vi "BypassControl.vi"(6 "Cutoff":dbl=0.15 format="%#_13g", 8 "MaxMotorChangeForward":dbl, 9 "MaxMotorChangeBackward":dbl, 10 "DesiredInput":dbl, 11 "CurrentInput":dbl) -> (2 "In range?":bool, 3 "SetMotor":dbl)   [LabVIEW 2015]
doc: "Skips motor values that are, for all intents and purposes, 0. This VI includes trapezoidal acceleration."
panel:
  in  "LoopTime":dbl
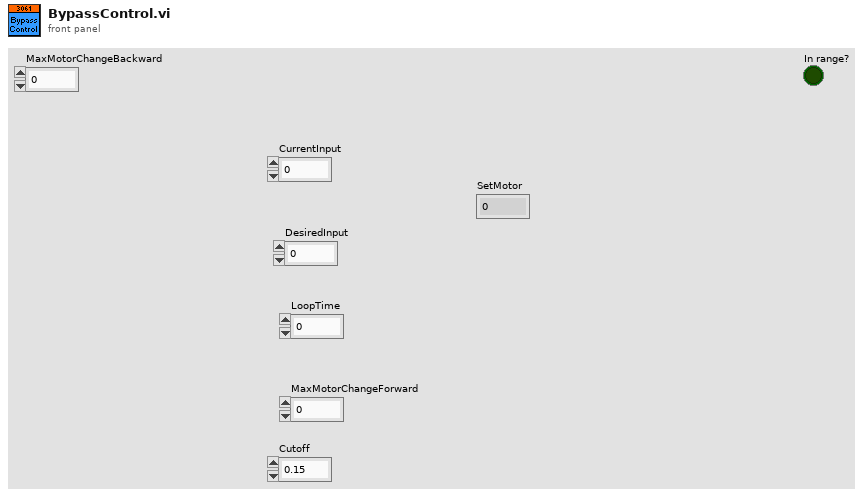
[diagram p1: front panel]
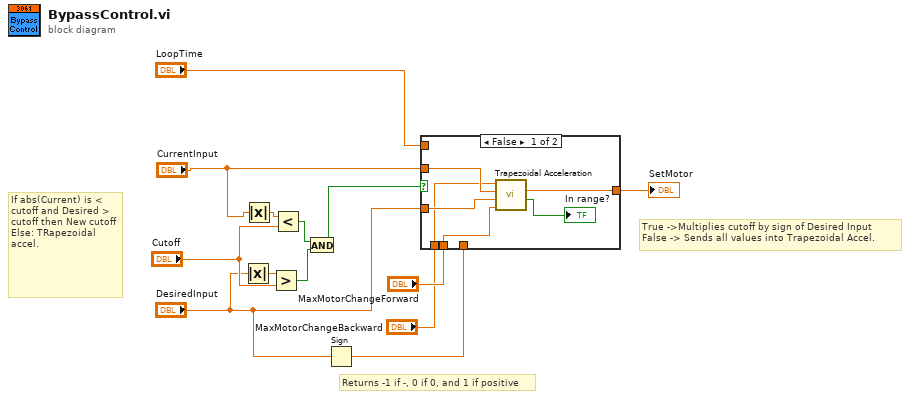
[diagram p0: block diagram]
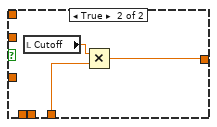
[diagram p2: hidden frame]
diagram:
  # "If abs(Current) is < cutoff and Desired > cutoff then New cutoff\nElse: TRapezoidal accel."
  # "True ->Multiplies cutoff by sign of Desired Input \nFalse -> Sends all values into Trapezoidal Accel."
  # "Returns -1 if -, 0 if 0, and 1 if positive"
  n1 = Absolute Value(x="DesiredInput") -> (abs(x)=w11:dbl)
  n2 = Absolute Value(x="CurrentInput") -> (abs(x)=w12:dbl)
  n3 = Greater?(x=w11, y="Cutoff") -> (0:w9:bool)
  n4 = Less?(x=w12, y="Cutoff") -> (x < y?=w10:bool)
  n5 = And(x=w10, y=w9) -> (x .and. y?=w8:bool)
  n6 = Sign(1:"DesiredInput") -> (0:w6:dbl)
  n7 = case shown="False" w8 {
    tunnel: "DesiredInput" -> [w18 _]
    tunnel: "CurrentInput" -> [w19 _]
    tunnel: [w17 w22] -> w5
    tunnel: w6 -> [_ w21]
    tunnel: "LoopTime" -> [_ _]
    tunnel: "MaxMotorChangeForward" -> [w16 _]
    tunnel: "MaxMotorChangeBackward" -> [w14 _]
    frame False {
      n8 = call "Trapezoidal Acceleration.vi"("MaxMotorChangeForward"=w16, "Desired"=w18, "Actual"=w19, "MaxMotorChangeBackward"=w14) -> ("In range?"=→"In range?":bool, "New Actual"=w17:dbl)  [unwired: 6 in]
    }
    frame True {
      n9 = local read "Cutoff"() -> (w20:dbl)
      n10 = Multiply(x=w20, y=w21) -> (x*y=w22:dbl)
    }
  }
  "SetMotor" <- w5
